vi "DFD Narrowband Filtering with State (Array).vi"(6 "state in":cluster{"state ":dbl[]}[](array[cluster]), 8 "error in (no error)":errorcluster, 10 "narrowband filter":T1 {"multirate filters"."mMRate_SumWl" min=1 max=32 step=1; "multirate filters"."mMRate_InputIwl" min=1 max=32 step=1; "multirate filters"."mMRate_GainWl" min=1 max=32 step=1; "multirate filters"."mMRate_OutputWl" min=1 max=32 step=1; "multirate filters"."mMRate_InputWl" min=1 max=32 step=1; "multirate filters"."mMRate_CoefWl" min=1 max=32 step=1; "multirate filters"."mMRate_Mode" items=["Default"=-1, "No Rate Change"=0, "Interpolation"=1, "Decimation"=2, "Interpolated"=3, "Rational"=4]}, 11 "signal in":dbl[](array[numeric])) -> (0 "error out":errorcluster, 3 "signal out":dbl[](array[numeric]), 4 "state out":cluster{"state ":dbl[]}[](array[cluster]))   [LabVIEW 2017, in "NI_DigFilterLicensed.lvlib"]
doc: "Filters a signal with a narrowband filter. You must specify the initial internal states in <B>state in</B> to generate an accurate output. Wire data to the <B>signal in</B> input to determine the polymorphic instance to use or manually select the instance."
uses:
  <vilib>/addons/Digital Filter Design/NI_DigFilterLicensed.lvlib
  <vilib>/addons/Digital Filter Design/_Objects.llb/DFD Narrowband Filter Obj.ctl
  <vilib>/addons/Digital Filter Design/_Objects.llb/DFD Multirate Filter Obj.ctl
  <vilib>/addons/Digital Filter Design/_Objects.llb/DFD Multirate Mode.ctl
  <vilib>/addons/Digital Filter Design/_Objects.llb/DFD Coef Norm Type.ctl
  <vilib>/addons/Digital Filter Design/_Objects.llb/DFD Round-off Mode.ctl
  <vilib>/addons/Digital Filter Design/_Objects.llb/DFD FXP MRate Multiply Mode.ctl
  <vilib>/addons/Digital Filter Design/Process.llb/DFD Integer Delay with State (Array).vi
  <vilib>/addons/Digital Filter Design/Multirate.llb/DFD NStage MRate Filtering with State (Array).vi
  <vilib>/addons/Digital Filter Design/NI_DigFilter_Process.lvlib
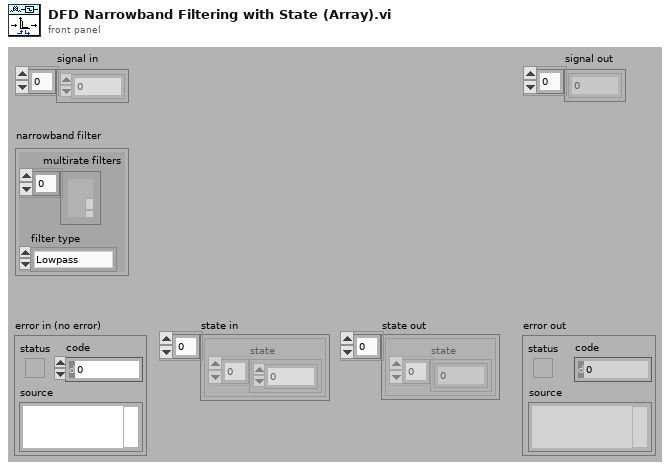
[diagram p1: front panel]
types:
  T1 = typedef "NI_DigFilterLicensed.lvlib/DFD Narrowband Filter Obj.ctl" = cluster{"multirate filters":T2[], "filter type":enum32{"Lowpass", "Highpass", "Bandpass", "Bandstop", "Wideband-Lowpass", "Wideband-Highpass"}}
  T2 = typedef "NI_DigFilterLicensed.lvlib/DFD Multirate Filter Obj.ctl" = cluster{"mMRate_Structure":enum16{"CIC", "FIR", "IIR", "Lattice"}, "mMRate_Mode":T3, "mMRate_Factor":i32, "mMRate_FIRParams":cluster{"mMRate_FIR_H":dbl[], "mMRate_FIR_IsNyquist?":bool, "mMRate_FIR_IsSymmetric?":bool}, "mMRate_CICParams":cluster{"mMRate_CIC_#Stage":i32, "mMRate_CIC_Lag":i32, "mMRate_CIC_Type":enum16{"Lowpass", "Highpass"}}, "mMRate_Order":i32, "mMRate_Version":string, "mMRate_Comments":string, "mMRate_RationalFactor":cluster{"mMRate_L":i32, "mMRate_M":i32}, "mMRate_Fs":dbl, "mMRate_Quantized?":bool, "mMRate_QFilterGain":dbl, "mMRate_CoefWl":i16, "mMRate_Scaling":cluster{"mMRate_ScaleByPowerOf2?":bool, "mMRate_ScaleType":T4}, "mMRate_InputWl":i16, "mMRate_OutputWl":i16, "mMRate_OutputMode":T5, "mMRate_MultMode":T6, "mMRate_BitPruning":bool, "mMRate_GainWl":i16, "mMRate_OutputFwl":i16, "mMRate_SumIwl":i16, "mMRate_InputIwl ":i16, "mMRate_SumWl":i16, "mMRate_CoefIwl":i16}
  T3 = typedef "NI_DigFilterLicensed.lvlib/DFD Multirate Mode.ctl" = i16
  T4 = typedef "NI_DigFilterLicensed.lvlib/DFD Coef Norm Type.ctl" = enum16{"No Norm", "Time Domain 1-Norm", "Time Domain 2-Norm", "Time Domain Inf-Norm"}
  T5 = typedef "NI_DigFilterLicensed.lvlib/DFD Round-off Mode.ctl" = enum16{"Nearest", "Truncation"}
  T6 = typedef "NI_DigFilterLicensed.lvlib/DFD FXP MRate Multiply Mode.ctl" = enum16{"Truncated", "Full"}
  T7 = enum32{"Lowpass", "Highpass", "Bandpass", "Bandstop", "Wideband-Lowpass", "Wideband-Highpass"}
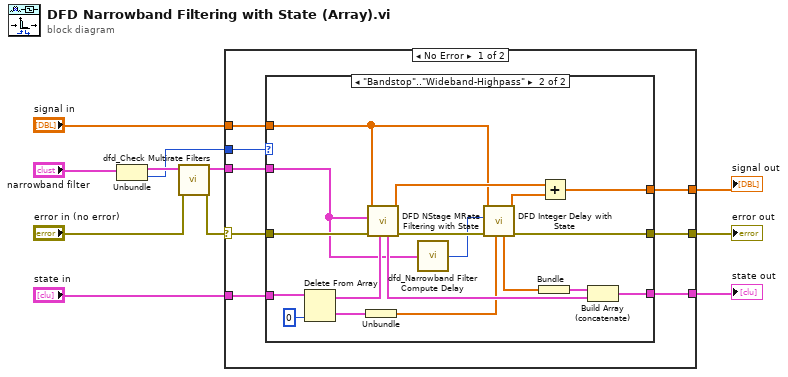
[diagram p0: block diagram]
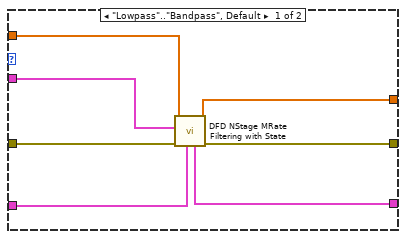
[diagram p2: hidden frame]
diagram:
  n1 = Unbundle("narrowband filter") -> ("multirate filters"=w6:T2[], "filter type"=w4:T7)
  n2 = call <vilib>:"dfd_Check Multirate Filters.vi"("error in (no error)"="error in (no error)", "multirate filters in"=w6) -> ("error out"=w1:errorcluster, "multirate filters out"=w3:T2[])  [unwired: 8 out]
  n3 = case shown="No Error" w1 {
    selector: w1 -> [w12 w45]
    tunnel: [w17 w45] -> w11
    tunnel: "signal in" -> [w19 _]
    tunnel: "state in" -> [w15 _]
    tunnel: [w18 _] -> w8
    tunnel: [w16 _] -> w7
    tunnel: w4 -> [w14 _]
    tunnel: w3 -> [w13 _]
    frame No Error {
      n4 = case shown="\"Bandstop\"..\"Wideband-Highpass\"" w14 {
        tunnel: w13 -> [w26 w30]
        tunnel: w19 -> [w20 w28]
        tunnel: [w25 w39] -> w18
        tunnel: [w24 w40] -> w17
        tunnel: [w21 w42] -> w16
        tunnel: w15 -> [w23 w34]
        tunnel: w12 -> [w22 w31]
        frame "Lowpass".."Bandpass", Default {
          n5 = call-poly <vilib>:"DFD NStage MRate Filtering with State.vi"("state in"=w23, "error in (no error)"=w22, "multirate filters"=w26, "signal in"=w20) -> ("error out"=w24:errorcluster, "signal out"=w21:dbl[], "state out"=w25:cluster{"state ":dbl[]}[])  [unwired: 5 out]
        }
        frame "Bandstop".."Wideband-Highpass" {
          n6 = Delete From Array(array=w34, index=0) -> (deleted portion=w36:cluster{"state ":dbl[]}, array with subset deleted=w32:cluster{"state ":dbl[]}[])  [unwired: 1 in]
          n7 = Unbundle(w36) -> ("state"=w33:dbl[])
          n8 = call-poly <vilib>:"DFD NStage MRate Filtering with State.vi"("state in"=w32, "error in (no error)"=w31, "multirate filters"=w30, "signal in"=w28) -> ("error out"=w43:errorcluster, "signal out"=w29:dbl[], "state out"=w44:cluster{"state ":dbl[]}[])  [unwired: 5 out]
          n9 = call <vilib>:"dfd_Narrowband Filter Compute Delay.vi"("multirate filters in"=w30) -> ("#sample"=w41:i32)
          n10 = call-poly <vilib>:"DFD Integer Delay with State.vi"("state in"=w33, "error in (no error)"=w43, "delay"=w41, "signal in"=w28) -> ("error out"=w40:errorcluster, "signal out"=w27:dbl[], "state out"=w38:dbl[])  [unwired: 5 out]
          n11 = Bundle("state out"=w38) -> (w37:cluster{"state out":dbl[]})  [unwired: 1 in]
          n12 = Add(x=w29, y=w27) -> (x+y=w42:dbl[])
          n13 = Build Array (concatenate)(w37, w44) -> (w39:cluster{"state ":dbl[]}[])
        }
      }
    }
    frame Error {
    }
  }
  "signal out" <- w7
  "error out" <- w11
  "state out" <- w8
